vi "Import.vi"(6 "Drop Position (0, 0)":cluster{"Left":i32, "Top":i32}, 7 "Application Refnum":refnum<vi>, 8 "error in (no error)":errorcluster, 9 "Copy to (\"VI\")":enum8{"VI", "Clipboard"}(ring), 10 "VI Snippet Path (.png)":path, 11 "VI Refnum (New VI)":refnum<vi>) -> (0 "error out":errorcluster, 2 "New VI?":bool, 3 "VI Refnum out":refnum<vi>)   [LabVIEW 2022 SP3, in "VI-Snippet.lvlib"]
doc: "Import the embedded VI within <b>VI Snippet Path (.png)</b>. Set <b>Copy to</b> as either <b>\"VI\"</b> to copy to a new VI or <b>\"Clipboard\"</b> to copy the VI Snippet content to the clipboard. If <b>VI Refnum</b> is NaN this creates a new VI. Otherwise, specify the <b>Drop Position</b> where to place content into an existing VI.\nNotes:\n- If <b>Copy to</b> is Clipboard, paste the snippet to a VI's block diagram.\n- The <b>Drop Position</b> has no effect for new VIs. \n- The <b>Copy to</b> <b>\"Clipboard\"</b> does not return a <b>VI Refnum out</b>."
uses:
  VI-Snippet.lvlib
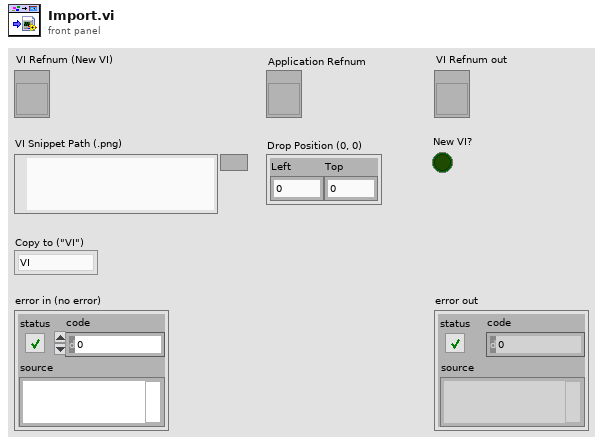
[diagram p1: front panel]
types:
  T1 = typedef "VI-Snippet.lvlib/Snippet.ctl" = cluster{"Image":cluster{"image type":i32, "image depth":i32, "image":u8[], "mask":u8[], "colors":u32[], "Rectangle":cluster{"left":i16, "top":i16, "right":i16, "bottom":i16}}, "niVI":string}
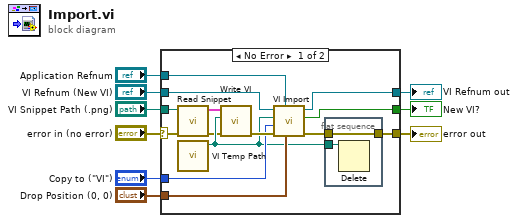
[diagram p0: block diagram]
diagram:
  n1 = case shown="No Error" "error in (no error)" {
    selector: "error in (no error)" -> [w22 w27]
    tunnel: "VI Snippet Path (.png)" -> [w21 _]
    tunnel: "VI Refnum (New VI)" -> [w18 w26]
    tunnel: "Drop Position (0, 0)" -> [w15 _]
    tunnel: [w23 w27] -> w8
    tunnel: [w13 w26] -> w6
    tunnel: [w12 _] -> w5
    tunnel: "Copy to (\"VI\")" -> [w16 _]
    tunnel: "Application Refnum" -> [w17 _]
    frame No Error {
      n2 = call "Read Snippet.vi"("error in (no error)"=w22, "VI Snippet (.png)"=w21) -> ("error out"=w10:errorcluster, "Snippet"=w20:T1)  [unwired: 8 in]
      n3 = call "VI Temp Path.vi"() -> ("Path (.vi)"=w11:path)  [unwired: 11 in]
      n4 = call "Write VI.vi"("error in (no error)"=w10, "VI Path (.vi)"=w11, "Snippet"=w20) -> ("error out"=w19:errorcluster)  [unwired: 8 in]
      n5 = call "VI Import.vi"("Drop Position (0, 0)"=w15, "Application Refnum"=w17, "error in (no error)"=w19, "Copy to (\"VI\")"=w16, "VI Path (.vi)"=w11, "VI Refnum in (NaN=New VI)"=w18) -> ("error out"=w14:errorcluster, "Created New VI?"=w12:bool, "VI Refnum out"=w13:refnum<vi>)  [unwired: 3 in]
      n6 = flat-sequence {
        tunnel: w11 -> [w25]
        tunnel: [w24] -> w23
        tunnel: w14 -> [w24]
        frame #0 {
          n7 = Delete(path (use dialog)=w25) -> ()  [unwired: 4 in, 3 out]
        }
      }
    }
    frame Error {
    }
  }
  "error out" <- w8
  "VI Refnum out" <- w6
  "New VI?" <- w5
